vi "Pid_v14.vi"() -> ()   [LabVIEW 2020]
panel:
  out "u - Comanda":dbl(graph)=49.999877814419186
  out "y - Iesirea":dbl(slide)=49.99941110945184 scale=40.0..60.0
  in  "stop":bool
  out "y":dbl=49.99941110945184
  out "u":dbl(slide)=49.999877814419186 scale=40.0..60.0
  out "y,r,u":cluster{"r-Set point":dbl, dbl, dbl}(graph)={"r-Set point"=49.99941110945184, 50.0, 49.999877814419186}
  in  "Kd":dbl(slide)=0.1111111111111111 scale=0.0..0.5
  in  "Kp":dbl(slide)=0.3508771929824561 scale=0.0..2.5
  in  "Ki":dbl(slide)=0.8888888888888888 scale=0.0..2.0
  in  "r - Set point":dbl(slide)=50.0 scale=40.0..60.0
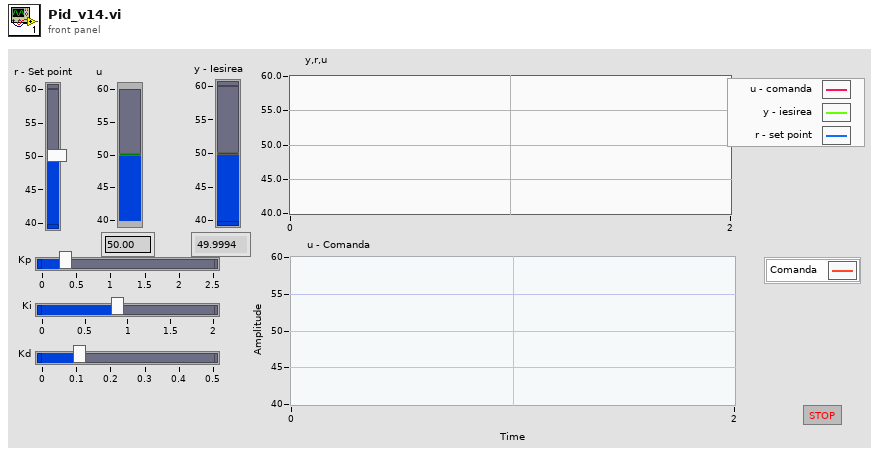
[diagram p1: front panel]
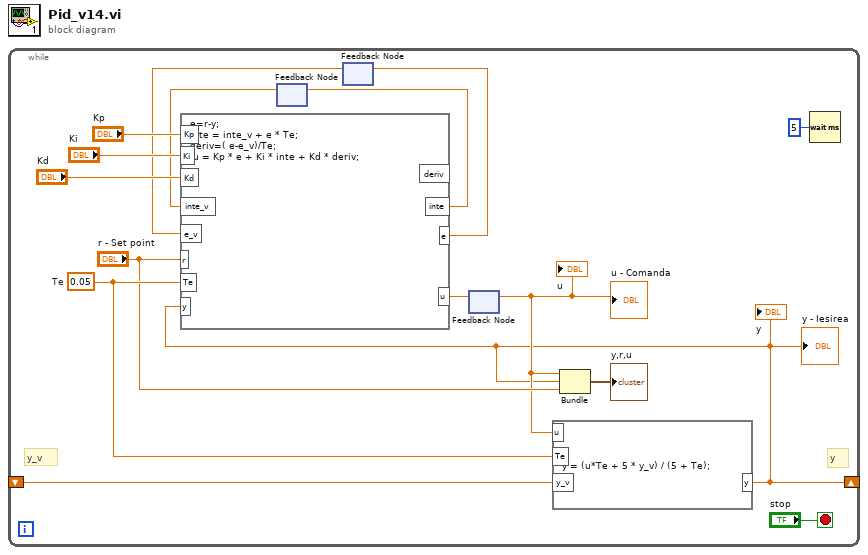
[diagram p0: block diagram]
diagram:
  n1 = while {
    shift-right: [w6] -> _
    shift-left: _ -> [w10]
    stop <- "stop" stop-if-true
    w9 = 0.05  # Te
    # "y_v"
    # "y"
    n2 = feedback #1() -> (w3:dbl)  [unwired: 1 in]
    n3 = feedback #2() -> (w1:dbl)  [unwired: 1 in]
    n4 = feedback #3() -> (w7:dbl)  [unwired: 1 in]
    "u" <- w7
    "u - Comanda" <- w7
    n5 = formula code="y = (u*Te + 5 * y_v) / (5 + Te);"("y_v"=w10, "u"=w7, "Te"=w9) -> ("y"=w6:dbl)
    "y" <- w6
    "y - Iesirea" <- w6
    n6 = formula code="e=r-y;\ninte = inte_v + e * Te;\nderiv=( e-e_v)/Te;\n u = Kp * e + Ki * inte + Kd * deriv;"("inte_v"=w3, "Te"=w9, "e_v"=w1, "Kp"="Kp", "Ki"="Ki", "Kd"="Kd", "r"="r - Set point", "y"=w6) -> ("inte"=w4:dbl, "u"=w11:dbl, "e"=w2:dbl)  [unwired: 1 out]
    n7 = feedback-in #1(w4) -> ()
    n8 = feedback-in #2(w2) -> ()
    n9 = feedback-in #3(w11) -> ()
    n10 = Bundle("u"=w7, "y"=w6, "r - Set point"="r - Set point") -> (→"y,r,u":cluster{"u":dbl, "y":dbl, "r - Set point":dbl})  [unwired: 1 in]
    n11 = Wait (ms)(milliseconds to wait=u32 5) -> ()  [unwired: 1 out]
  }
